vi "Up Hole PRESSURE_CAL 2016.vi"(4 "Pressure Offset":dbl format="%.2f", 6 "Descriptions":string[](array[string]), 7 "Array in":refnum<k24>[](array[refnum]), 9 "Pressure \nSlope":dbl=24.27199935913086 format="%.2f", 10 "Sensor Cluster":T1, 11 "Prompt_IN":string) -> (3 "PRESSURE\nFt of water":dbl format="%.2f", 5 "Array out":refnum<k24>[](array[refnum]))   [LabVIEW 2016]
uses:
  Waterloo DAQ/controls/MCC DAQ Readings.ctl
  C:/Program Files (x86)/National Instruments/LabVIEW 2016/vi.lib/ULx/ULx_LV.dll
panel:
  out "Setup_instructions":string
  in  "OK Button":bool
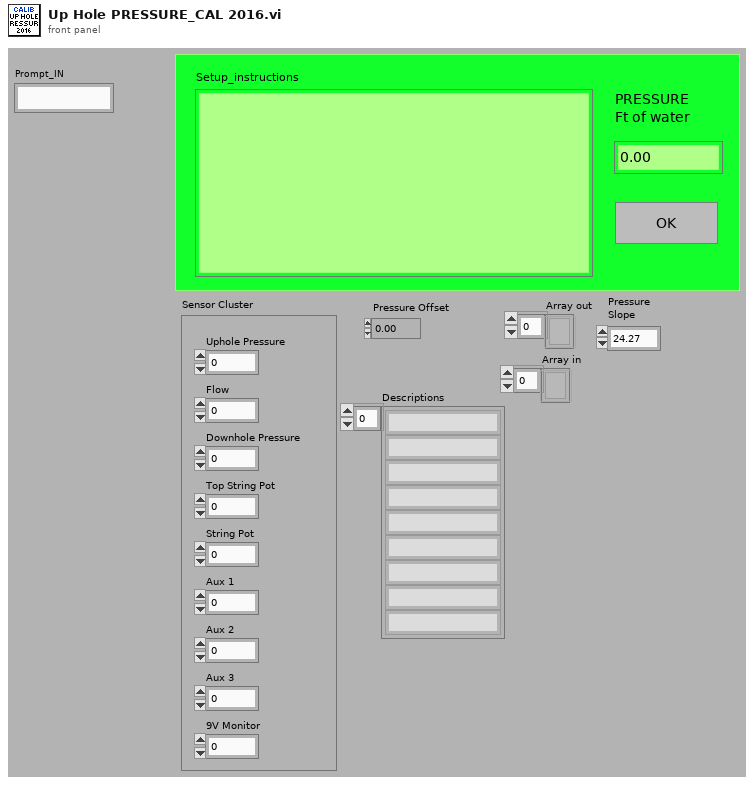
[diagram p1: front panel]
types:
  T1 = typedef "MCC DAQ Readings.ctl" = cluster{"Uphole Pressure":dbl, "Flow":dbl, "Downhole Pressure":dbl, "Top String Pot":dbl, "String Pot":dbl, "Aux 1":dbl, "Aux 2":dbl, "Aux 3":dbl, "9V Monitor":dbl}
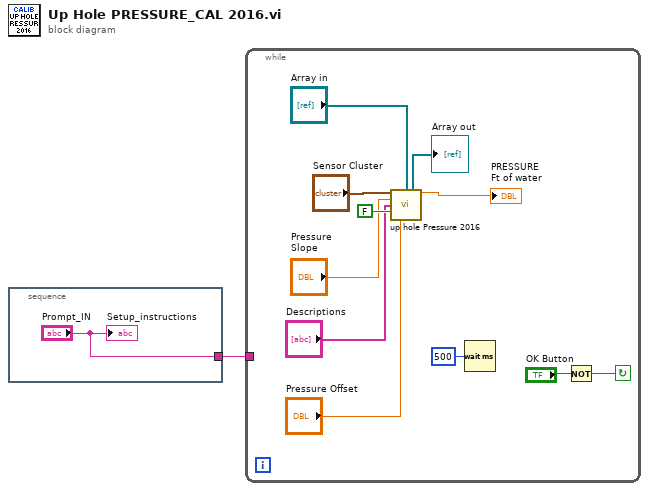
[diagram p0: block diagram]
diagram:
  n1 = stacked-sequence {
    tunnel: ["Prompt_IN"] -> w1
    frame #0 {
      "Setup_instructions" <- "Prompt_IN"
    }
  }
  n2 = while {
    tunnel: w1 -> [_]
    stop <- w11 continue-if-true
    n3 = call "up hole Pressure 2016.vi"("Sensor Cluster"="Sensor Cluster", "Pressure Offset"="Pressure Offset", "Array in"="Array in", "Pressure \nSlope"="Pressure \nSlope", "Descriptions"="Descriptions", "Zero Pressure\n(F = leave as is)"=FALSE ("Zero Pressure\n(F = leave as is)")) -> ("Array out"=→"Array out":refnum<k24>[], "Uphole Pressure"=→"PRESSURE\nFt of water":dbl)  [unwired: 6 in, 2 out]
    n4 = Wait (ms)(milliseconds to wait=u32 500) -> ()  [unwired: 1 out]
    n5 = Not(x="OK Button") -> (.not. x?=w11:bool)
  }
